vi "AlliGator Convert Phasor Value to Phasor Image Coordinates (N).vi"(8 "Phasor Plot Reference Points":T1, 10 "Phasor s":dbl[](array[numeric]), 11 "Phasor g":dbl[](array[numeric])) -> (2 "Phasor Plot y":i32[](array[numeric]), 3 "Phasor Plot x":i32[](array[numeric]))   [LabVIEW 2021, in "AlliGator Phasor Plot.lvlib"]
doc: "Converts array of phasor values to the corresponding array of Phasor Plot image coordinates."
uses:
  AlliGator Phasor Plot.lvlib
  Phasor Ratio/AlliGator Phasor Plot Reference Points.ctl
  Phasor Ratio/AlliGator Phasor Ratio.lvlib
panel:
  # "see the AlliGator License on the block diagram (Ctrl+E or Window:Show Block Diagram)"
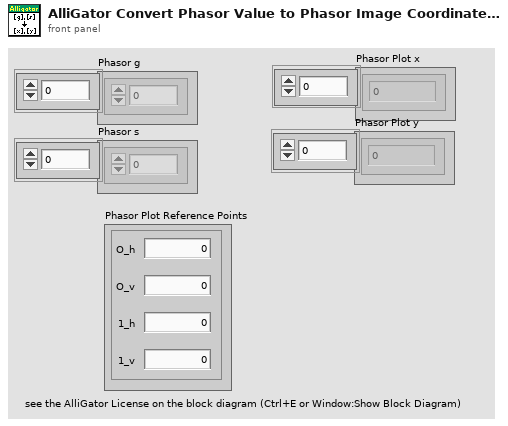
[diagram p1: front panel]
types:
  T1 = typedef "AlliGator Phasor Ratio.lvlib/AlliGator Phasor Plot Reference Points.ctl" = cluster{"O_h":dbl, "O_v":dbl, "1_h":dbl, "1_v":dbl}
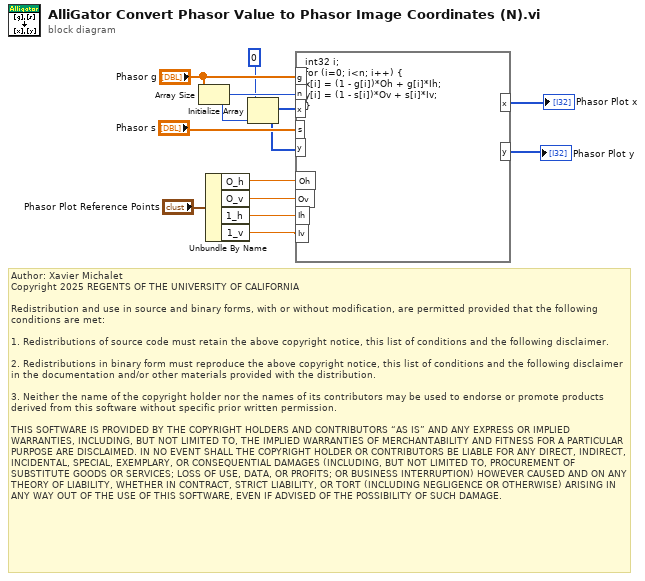
[diagram p0: block diagram]
diagram:
  # "Author: Xavier Michalet\nCopyright 2025 REGENTS OF THE UNIVERSITY OF CALIFORNIA\n\nRedistribution and use in source and binary forms, with or without modification, are permitted provided that the following conditions are met:\n\n1. Redistributions of source code must retain the above copyright notice, this list of conditions and the following disclaimer.\n\n2. Redistributions in binary form must reproduce the above copyright notice, this list of conditions and the following disclaimer in the documentation and/or other materials provided with the distribution.\n\n3. Neither the name of the copyright holder nor the names of its contributors may be used to endorse or promote products derived from this software without specific prior written permission.\n\nTHIS SOFTWARE IS PROVIDED BY THE COPYRIGHT HOLDERS AND CONTRIBUTORS “AS IS” AND ANY EXPRESS OR IMPLIED WARRANTIES, INCLUDING, BUT NOT LIMITED TO, THE IMPLIED WARRANTIES OF MERCHANTABILITY AND FITNESS FOR A PARTICULAR PURPOSE ARE DISCLAIMED. IN NO EVENT SHALL THE COPYRIGHT HOLDER OR CONTRIBUTORS BE LIABLE FOR ANY DIRECT, INDIRECT, INCIDENTAL, SPECIAL, EXEMPLARY, OR CONSEQUENTIAL DAMAGES (INCLUDING, BUT NOT LIMITED TO, PROCUREMENT OF SUBSTITUTE GOODS OR SERVICES; LOSS OF USE, DATA, OR PROFITS; OR BUSINESS INTERRUPTION) HOWEVER CAUSED AND ON ANY THEORY OF LIABILITY, WHETHER IN CONTRACT, STRICT LIABILITY, OR TORT (INCLUDING NEGLIGENCE OR OTHERWISE) ARISING IN ANY WAY OUT OF THE USE OF THIS SOFTWARE, EVEN IF ADVISED OF THE POSSIBILITY OF SUCH DAMAGE."
  n1 = Array Size(array="Phasor g") -> (size(s)=w3:i32)
  n2 = Unbundle By Name("Phasor Plot Reference Points") -> ("O_h"=w11:dbl, "O_v"=w10:dbl, "1_h"=w9:dbl, "1_v"=w8:dbl)
  n3 = Initialize Array(0 ("Phasor Plot x"), w3) -> (w1:i32[])
  n4 = formula code="int32 i;\nfor (i=0; i<n; i++) {\nx[i] = (1 - g[i])*Oh + g[i]*Ih;\ny[i] = (1 - s[i])*Ov + s[i]*Iv;\n}"("g"="Phasor g", "s"="Phasor s", "Oh"=w11, "Ov"=w10, "Ih"=w9, "Iv"=w8, "n"=w3, "x"=w1, "y"=w1) -> ("x"=→"Phasor Plot x":i32[], "y"=→"Phasor Plot y":i32[])
